vi "E3644A_Config.vi"(0 "VISA resource name":refnum<visa-resource-name>, 2 "Current Limit (A)":dbl=0.01 format="%.2p", 3 "Voltage Level (V)":dbl=5.0 format="%.2p", 5 "error in (no error)":errorcluster, 8 "ID Query (T: Query)":bool=TRUE, 10 "Reset Device (T: Reset)":bool=TRUE, 11 "Output Enabled (F: Off)":bool, 12 "Measure Enable ?":bool) -> (16 "Measurement":dbl format="%.2p", 19 "error out":errorcluster)   [LabVIEW 2016]
uses:
  <userlib>/_TI-LA/Instr Drivers/Power Supply/E364x/Driver/Base/Agilent E364X Series.lvlib
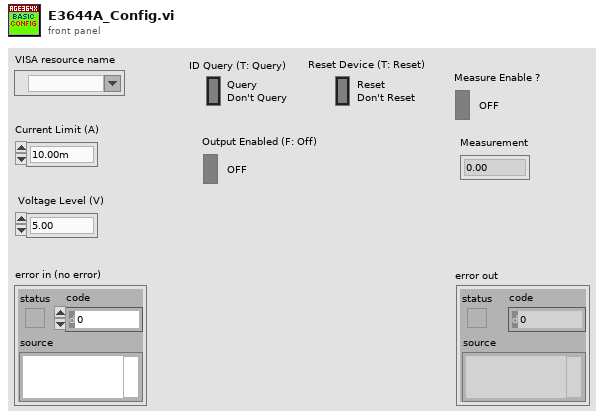
[diagram p1: front panel]
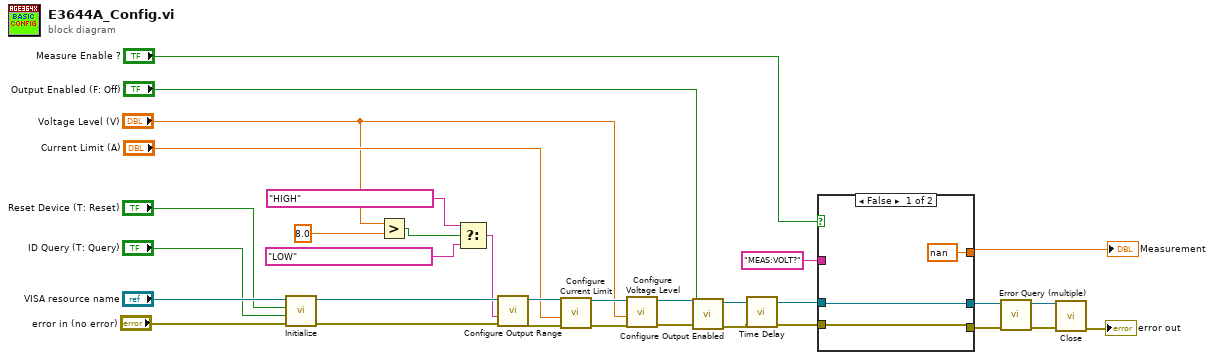
[diagram p0: block diagram]
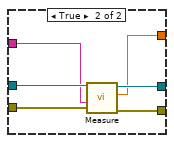
[diagram p2: hidden frame]
diagram:
  n1 = call <userlib>:"Initialize.vi"("error in (no error)"="error in (no error)", "ID Query (T: Query)"="ID Query (T: Query)", "Reset Device (T: Reset)"="Reset Device (T: Reset)", "VISA resource name"="VISA resource name") -> ("error out"=w19:errorcluster, "VISA resource name out"=w20:refnum<visa-resource-name>)  [unwired: 6 in]
  n2 = Greater?(x="Voltage Level (V)", y=8.0) -> (0:w8:bool)
  n3 = Select(t="HIGH" ("Range (High Voltage / Low Current)"), s=w8, f="LOW" ("Range (High Voltage / Low Current)")) -> (s? t:f=w11:string)
  n4 = call <userlib>:"Configure Output Range.vi"("error in (no error)"=w19, "Range (High Voltage / Low Current)"=w11, "VISA resource name"=w20) -> ("error out"=w30:errorcluster, "VISA resource name out"=w31:refnum<visa-resource-name>)  [unwired: 7 in]
  n5 = call <userlib>:"Configure Current Limit.vi"("error in (no error)"=w30, "Current Limit (0.0 Amps)"="Current Limit (A)", "VISA resource name"=w31) -> ("error out"=w29:errorcluster, "VISA resource name out"=w28:refnum<visa-resource-name>)  [unwired: 7 in]
  n6 = call <userlib>:"Configure Voltage Level.vi"("error in (no error)"=w29, "Level (0.0 Volts)"="Voltage Level (V)", "VISA resource name"=w28) -> ("error out"=w26:errorcluster, "VISA resource name out"=w27:refnum<visa-resource-name>)  [unwired: 7 in]
  n7 = call <userlib>:"Configure Output Enabled.vi"("error in (no error)"=w26, "Output Enabled (F: Off)"="Output Enabled (F: Off)", "VISA resource name"=w27) -> ("error out"=w24:errorcluster, "VISA resource name out"=w25:refnum<visa-resource-name>)  [unwired: 7 in]
  n8 = call "Time Delay"("error in (no error)"=w24) -> ("error out"=w23:errorcluster)  [unwired: 10 in]
  n9 = case shown="False" "Measure Enable ?" {
    tunnel: w25 -> [w33 w40]
    tunnel: [w32 w39] -> w3
    tunnel: [w33 w38] -> w4
    tunnel: w23 -> [w32 w37]
    tunnel: [nan ("Measurement") w36] -> w13
    tunnel: "MEAS:VOLT?" ("Measurement Type (Voltage)") -> [_ w35]
    frame False {
    }
    frame True {
      n10 = call <userlib>:"Measure.vi"("error in (no error)"=w37, "Measurement Type (Voltage)"=w35, "VISA resource name"=w40) -> ("error out"=w39:errorcluster, "Measurement"=w36:dbl, "VISA resource name out"=w38:refnum<visa-resource-name>)  [unwired: 6 in]
    }
  }
  "Measurement" <- w13
  n11 = call <userlib>:"Error Query (multiple).vi"("error in (no error)"=w3, "VISA resource name"=w4) -> ("error out"=w2:errorcluster, "VISA resource name out"=w1:refnum<visa-resource-name>)  [unwired: 6 in, 2 out]
  n12 = call <userlib>:"Close.vi"("error in (no error)"=w2, "VISA resource name"=w1) -> ("error out"=→"error out":errorcluster)  [unwired: 9 in]
